vi "OPC_celda.vi"(0 "power":bool, 1 "Pulp ref":u16, 3 "water ref":i32, 4 "Setpoint Flujometro":u16, 5 "queue":refnum<queue>, 7 "error in (no error)":errorcluster, 9 "Gang ref":u16 max=100, 10 "Gas holdup":dbl, 11 "Altura capa de espuma":dbl, 12 "Record":bool, 13 "emergency  \nopen/close \nvalve":bool, 14 "Procesar datos\nen Matlab":bool, 15 "iteration":i32, 17 "ref pulp":dbl) -> (20 "output cluster":T1, 25 "queue out":refnum<queue>, 27 "error out":errorcluster)   [LabVIEW 2013]
uses:
  medidas.ctl
  bus to create file.ctl
  data simulation bus.ctl
  VoltElectrodo.ctl
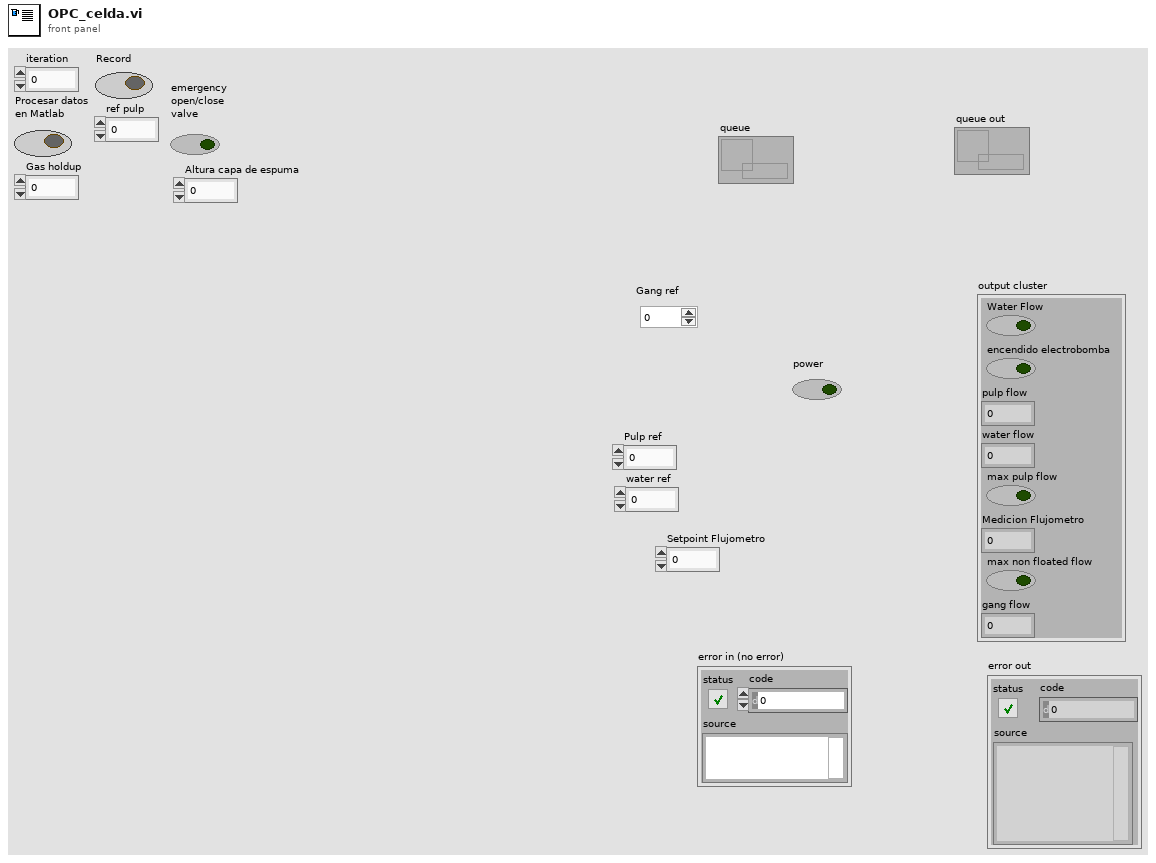
[diagram p1: front panel]
types:
  T1 = typedef "medidas.ctl" = cluster{"Water Flow":bool, "encendido electrobomba":bool, "pulp flow":dbl, "water flow":dbl, "max pulp flow":bool, "Medicion Flujometro":u16, "max non floated flow ":bool, "gang flow":dbl}
  T2 = typedef "data simulation bus.ctl" = cluster{"Flujo pulpa ":dbl, "Flujo agua lavado":dbl, "Flujo aire":dbl, "Flujo relave":dbl, "Altura capa de espuma":dbl, "Gas holdup":dbl, "% apertura valvula aire":dbl, "ref pulp":dbl}
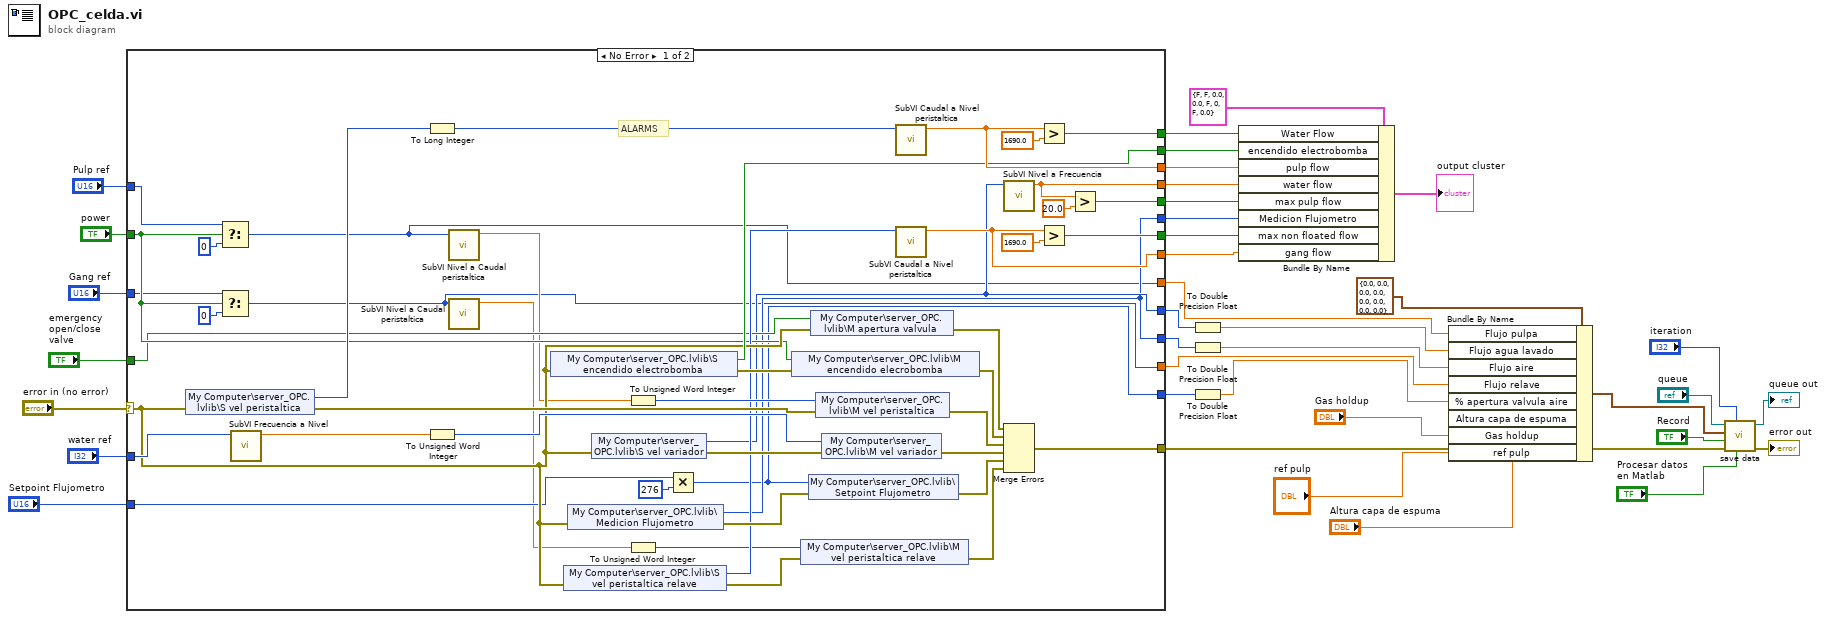
[diagram p0: block diagram]
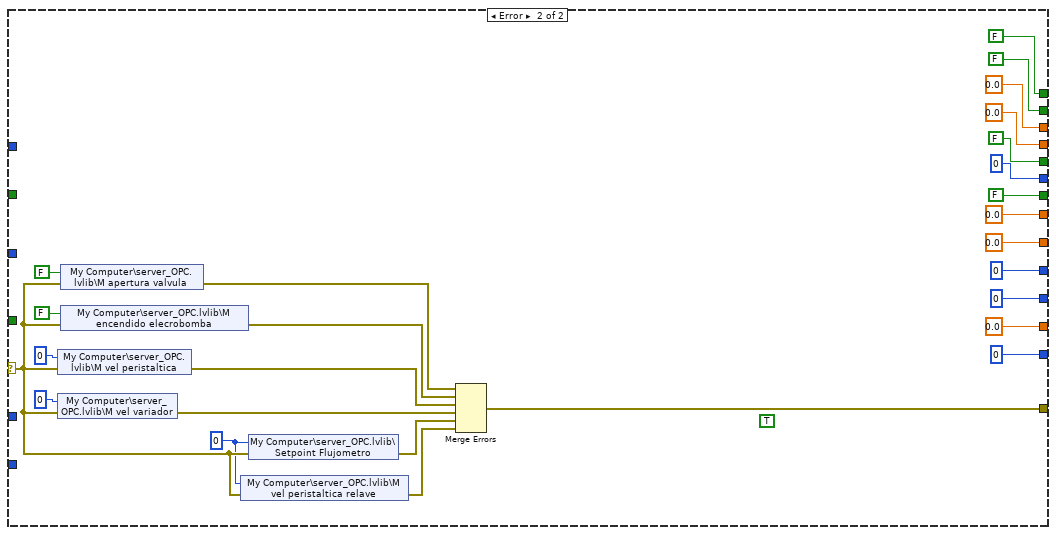
[diagram p2: hidden frame]
diagram:
  n1 = case shown="No Error" "error in (no error)" {
    selector: "error in (no error)" -> [w57 w92]
    tunnel: "power" -> [w52 _]
    tunnel: "Pulp ref" -> [w83 _]
    tunnel: [w59 w100] -> w20
    tunnel: "water ref" -> [w82 _]
    tunnel: "Setpoint Flujometro" -> [w45 _]
    tunnel: [w81 0.0 ("Numeric")] -> w31
    tunnel: [w80 0.0 ("Numeric out")] -> w30
    tunnel: [w79 FALSE] -> w29
    tunnel: [w78 FALSE] -> w28
    tunnel: [w42 u16 0 ("UInt16")] -> w27
    tunnel: [w77 FALSE ("Boolean")] -> w26
    tunnel: [w53 FALSE] -> w24
    tunnel: "Gang ref" -> [w51 _]
    tunnel: [w48 0.0 ("Numeric out")] -> w22
    tunnel: "emergency  \nopen/close \nvalve" -> [w47 _]
    tunnel: [w40 0.0 ("Numeric")] -> w17
    tunnel: [w43 u16 0 ("UInt16")] -> w16
    tunnel: [w42 u16 0 ("UInt16")] -> w15
    tunnel: [w39 0.0 ("Numeric")] -> w14
    tunnel: [w41 u16 0] -> w12
    frame No Error {
      # "ALARMS"
      n2 = shared-variable "My Computer\\server_OPC.lvlib\\S vel peristaltica"(error in=w57) -> (w76:u16, error out=w72:errorcluster)
      n3 = Select(t=w83, s=w52, f=u16 0) -> (s? t:f=w40:u16)
      n4 = Select(t=w51, s=w52, f=u16 0) -> (s? t:f=w39:u16)
      n5 = call "SubVI Frecuencia a Nivel.vi"("Pulp ref"=w82) -> ("Numeric"=w75:dbl)  [unwired: 10 in]
      n6 = To Long Integer(number=w76) -> (32bit integer=w70:i32)
      n7 = To Unsigned Word Integer(number=w75) -> (unsigned 16bit integer=w68:u16)
      n8 = call "SubVI Nivel a Caudal peristaltica.vi"("UInt16"=w40) -> ("Numeric"=w44:dbl)  [unwired: 10 in]
      n9 = call "SubVI Nivel a Caudal peristaltica.vi"("UInt16"=w39) -> ("Numeric"=w38:dbl)  [unwired: 10 in]
      n10 = shared-variable "My Computer\\server_OPC.lvlib\\S encendido electrobomba"(error in=w57) -> (w77:bool, error out=w71:errorcluster)
      n11 = shared-variable "My Computer\\server_OPC.lvlib\\S vel peristaltica relave"(error in=w57) -> (w55:u16, error out=w56:errorcluster)
      n12 = shared-variable "My Computer\\server_OPC.lvlib\\Medicion Flujometro"(error in=w57) -> (w42:u16, error out=w74:errorcluster)
      n13 = shared-variable "My Computer\\server_OPC.lvlib\\S vel variador"(error in=w57) -> (w43:u16, error out=w73:errorcluster)
      n14 = To Unsigned Word Integer(number=w44) -> (unsigned 16bit integer=w69:u16)
      n15 = To Unsigned Word Integer(number=w38) -> (unsigned 16bit integer=w49:u16)
      n16 = Multiply(x=w45, y=u16 276) -> (x*y=w41:u16)
      n17 = shared-variable "My Computer\\server_OPC.lvlib\\M encendido elecrobomba"(w52, error in=w71) -> (error out=w61:errorcluster)
      n18 = shared-variable "My Computer\\server_OPC.lvlib\\M vel peristaltica relave"(w49, error in=w56) -> (error out=w58:errorcluster)
      n19 = shared-variable "My Computer\\server_OPC.lvlib\\Setpoint Flujometro"(w41, error in=w74) -> (error out=w64:errorcluster)
      n20 = shared-variable "My Computer\\server_OPC.lvlib\\M apertura valvula"(w47, error in=w57) -> (error out=w60:errorcluster)
      n21 = shared-variable "My Computer\\server_OPC.lvlib\\M vel peristaltica"(w69, error in=w72) -> (error out=w62:errorcluster)
      n22 = shared-variable "My Computer\\server_OPC.lvlib\\M vel variador"(w68, error in=w73) -> (error out=w63:errorcluster)
      n23 = call "SubVI Caudal a Nivel peristaltica.vi"("Numeric in"=w70) -> ("Numeric out"=w80:dbl)  [unwired: 10 in]
      n24 = call "SubVI Caudal a Nivel peristaltica.vi"("Numeric in"=w55) -> ("Numeric out"=w48:dbl)  [unwired: 10 in]
      n25 = call "SubVI Nivel a Frecuencia.vi"("UInt16"=w43) -> ("Numeric"=w81:dbl)  [unwired: 10 in]
      n26 = Merge Errors(w60, w61, w62, w63, w64, w58) -> (w59:errorcluster)
      n27 = Greater?(x=w80, y=1690.0) -> (0:w79:bool)
      n28 = Greater?(x=w48, y=1690.0) -> (0:w53:bool)
      n29 = Greater?(x=w81, y=20.0) -> (0:w78:bool)
    }
    frame Error {
      (unwired) TRUE
      w91 = u16 0 ("Setpoint Flujometro")
      n30 = shared-variable "My Computer\\server_OPC.lvlib\\M vel peristaltica"(u16 0 ("M vel peristaltica"), error in=w92) -> (error out=w102:errorcluster)
      n31 = shared-variable "My Computer\\server_OPC.lvlib\\M vel variador"(u16 0 ("M vel variador"), error in=w92) -> (error out=w103:errorcluster)
      n32 = shared-variable "My Computer\\server_OPC.lvlib\\M apertura valvula"(FALSE ("M apertura valvula"), error in=w92) -> (error out=w108:errorcluster)
      n33 = shared-variable "My Computer\\server_OPC.lvlib\\M encendido elecrobomba"(FALSE ("M encendido elecrobomba"), error in=w92) -> (error out=w101:errorcluster)
      n34 = shared-variable "My Computer\\server_OPC.lvlib\\M vel peristaltica relave"(w91, error in=w92) -> (error out=w93:errorcluster)
      n35 = shared-variable "My Computer\\server_OPC.lvlib\\Setpoint Flujometro"(w91, error in=w92) -> (error out=w104:errorcluster)
      n36 = Merge Errors(w108, w101, w102, w103, w104, w93) -> (w100:errorcluster)
    }
  }
  n37 = To Double Precision Float(number=w16) -> (double precision float=w13:dbl)
  n38 = To Double Precision Float(number=w15) -> (double precision float=w10:dbl)
  n39 = To Double Precision Float(number=w12) -> (double precision float=w11:dbl)
  n40 = Bundle By Name(cluster=T1 {"Water Flow"=FALSE, "encendido electrobomba"=FALSE, "pulp flow"=0.0, "water flow"=0.0, "max pulp flow"=FALSE, "Medicion Flujometro"=0, "max non floated flow "=FALSE, "gang flow"=0.0}, "Water Flow"=w29, "encendido electrobomba"=w26, "pulp flow"=w30, "water flow"=w31, "max pulp flow"=w28, "Medicion Flujometro"=w27, "max non floated flow"=w24, "gang flow"=w22) -> (→"output cluster":T1)
  n41 = Bundle By Name(cluster=T2 {"Flujo pulpa "=0.0, "Flujo agua lavado"=0.0, "Flujo aire"=0.0, "Flujo relave"=0.0, "Altura capa de espuma"=0.0, "Gas holdup"=0.0, "% apertura valvula aire"=0.0, "ref pulp"=0.0} ("data save DAQ"), "Flujo pulpa"=w17, "Flujo agua lavado"=w13, "Flujo aire"=w10, "Flujo relave"=w14, "% apertura valvula aire"=w11, "Altura capa de espuma"="Altura capa de espuma", "Gas holdup"="Gas holdup", "ref pulp"="ref pulp") -> (w19:T2)
  n42 = call "save data.vi"("Procesar datos\nen Matlab"="Procesar datos\nen Matlab", "iteration"="iteration", "error in (no error)"=w20, "Record"="Record", "data save DAQ"=w19, "queue"="queue") -> ("error out"=→"error out":errorcluster, "queue out"=→"queue out":refnum<queue>)  [unwired: 4 in]
